vi "CPU_Overload.vi"(2 "Sample dt":i64, 3 "Iteration Duration":i64) -> (0 "CPU_Overload?":bool, 1 "DP_Overhead":i64)   [LabVIEW 2024]
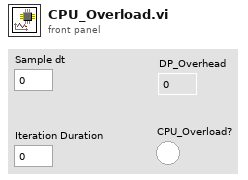
[diagram p1: front panel]
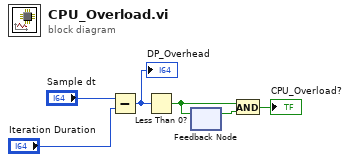
[diagram p0: block diagram]
diagram:
  n1 = Subtract(x="Sample dt", y="Iteration Duration") -> (x-y=w4:i64)
  "DP_Overhead" <- w4
  n2 = Less Than 0?(x=w4) -> (x < 0?=w2:bool)
  n3 = feedback-in #1(w2) -> ()
  n4 = feedback #1() -> (w1:bool)  [unwired: 1 in]
  n5 = And(x=w2, y=w1) -> (x .and. y?=→"CPU_Overload?":bool)
